vi "Set Power Cells.vi"(10 "Array":bool[](array[boolean])=[FALSE, FALSE, FALSE, FALSE, FALSE, FALSE], 11 "Knob in":refnum<vi>) -> (3 "Knob out":refnum<vi>)   [LabVIEW 2019]
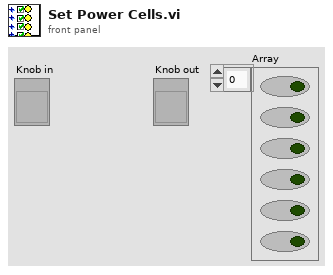
[diagram p1: front panel]
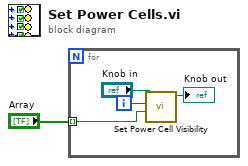
[diagram p0: block diagram]
diagram:
  n1 = for {
    tunnel: "Array" -> [w4] mode=indexing
    i -> [w5]
    n2 = call "Set Power Cell Visibility.vi"("Show"=w4, "Ball Slot"=w5, "Knob in"="Knob in") -> ("Knob out"=→"Knob out":refnum<vi>)  [unwired: 8 in]
  }
